vi "main.vi"(4 "force_read?":bool, 6 "custom_path":path, 7 "command":T1=enum."read_config", 8 "error in (no error)":errorcluster, 11 "config in":T2) -> (0 "error out":errorcluster, 3 "config out":T2)   [LabVIEW 2015, in "lv-config-json.lvlib"]
doc: "This VI is able to read/write configuration from all the associated modules defined in the master data cluster. It also acts as a functional global/data store in the event that no data has changed since the last write. It will self-initialize and well set an internal flag in the event an error is encountered when reading. If no command is provided, it will default to the read command."
uses:
  lv-config-json.lvlib
  public/_controls/configuration.ctl
  public/_controls/command.ctl
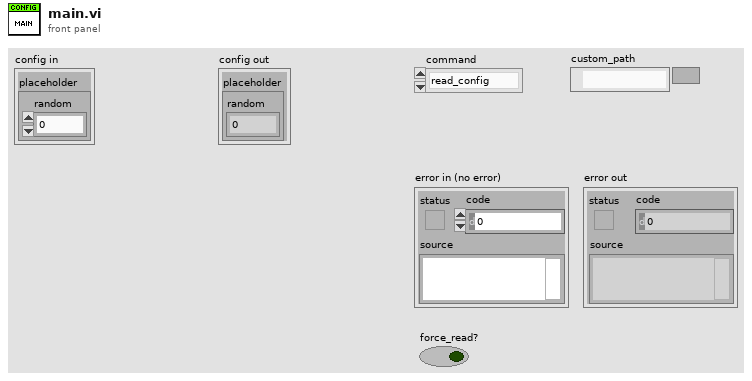
[diagram p1: front panel]
types:
  T1 = typedef "lv-config-json.lvlib/command.ctl" = enum16{"<commands>", "read_config", "write_config", "write_placeholder"}
  T2 = typedef "lv-config-json.lvlib/configuration.ctl" = cluster{"placeholder":cluster{"random":dbl}}
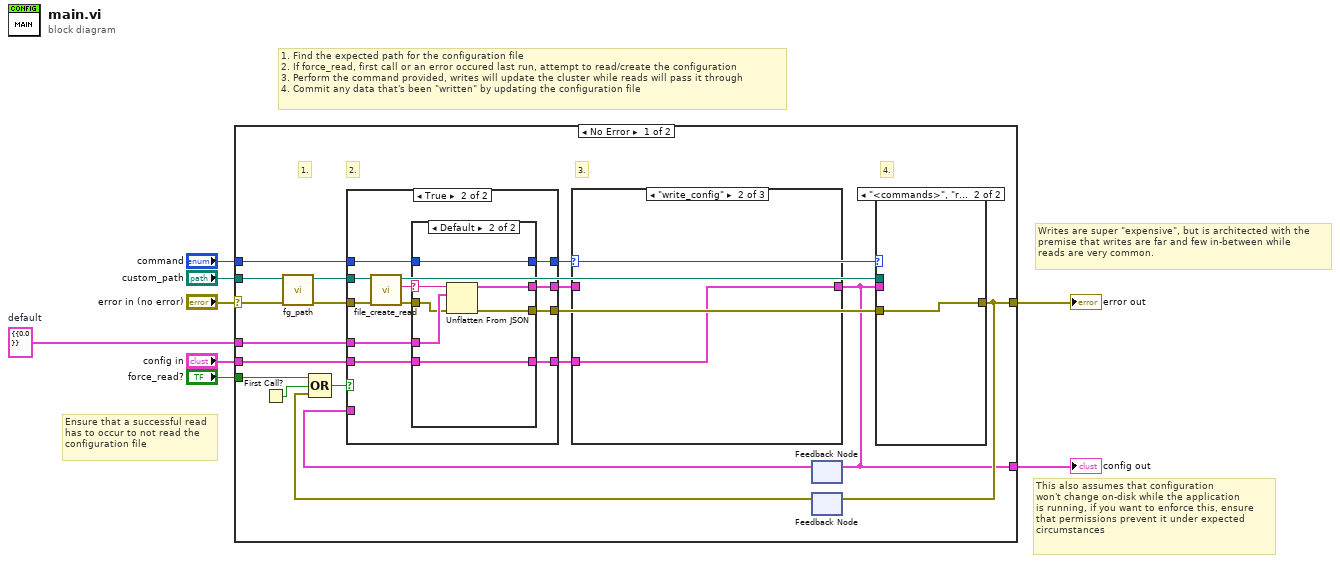
[diagram p0: block diagram]
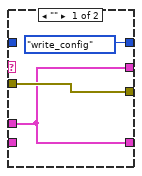
[diagram p3: hidden frame]
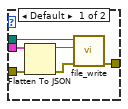
[diagram p4: hidden frame]
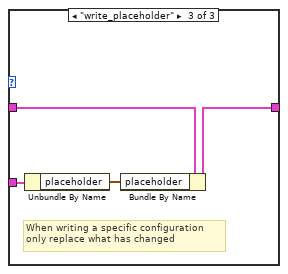
[diagram p6: hidden frame]
diagram:
  w1 = T2 {"placeholder"={"random"=0.0}}  # default
  # "This also assumes that configuration\nwon't change on-disk while the application\nis running, if you want to enforce this, ensure\nthat permissions prevent it under expected\ncircumstances"
  # "1. Find the expected path for the configuration file\n2. If force_read, first call or an error occured last run, attempt to read/create the configuration\n3. Perform the command provided, writes will update the cluster while reads will pass it through\n4. Commit any data that's been \"written\" by updating the configuration file"
  # "Writes are super \"expensive\", but is architected with the\npremise that writes are far and few in-between while\nreads are very common."
  # "Ensure that a successful read\nhas to occur to not read the\nconfiguration file"
  n1 = case shown="No Error" "error in (no error)" {
    selector: "error in (no error)" -> [w23 w65]
    tunnel: "command" -> [w13 _]
    tunnel: [w25 w65] -> w4
    tunnel: "config in" -> [w11 _]
    tunnel: "custom_path" -> [w22 _]
    tunnel: [w15 _] -> w3
    tunnel: "force_read?" -> [w20 _]
    tunnel: w1 -> [w16 _]
    frame No Error {
      # "4."
      # "3."
      # "2."
      # "1."
      n2 = First Call?() -> (First Call?: T/F=w21:bool)
      n3 = call "fg_path.vi"("error in (no error)"=w23, "custom_path"=w22) -> ("error out"=w17:errorcluster, "config_working"=w14:path)  [unwired: 8 in]
      n4 = feedback #1() -> (w18:T2)  [unwired: 1 in]
      n5 = feedback #2() -> (w24:errorcluster)  [unwired: 1 in]
      n6 = Compound Arithmetic op=OR(w20, w21, w24) -> (w19:bool)
      n7 = case shown="True" w19 {
        tunnel: w18 -> [w30 _]
        tunnel: w17 -> [w29 w39]
        tunnel: w14 -> [_ w40]
        tunnel: [w29 w37] -> w26
        tunnel: w16 -> [_ w41]
        tunnel: w13 -> [w28 w36]
        tunnel: [w28 w35] -> w12
        tunnel: w11 -> [w27 w34]
        tunnel: [w27 w33] -> w10
        tunnel: [w30 w32] -> w9
        frame False {
        }
        frame True {
          n8 = call "file_create_read.vi"("error in (no error)"=w39, "config_path"=w40) -> ("error out"=w38:errorcluster, "string"=w31:string)  [unwired: 8 in]
          n9 = case shown="Default" w31 {
            selector: w31 -> [_ w48]
            tunnel: w41 -> [w42 w51]
            tunnel: [w42 w50] -> w32
            tunnel: w38 -> [w44 w49]
            tunnel: [w44 w47] -> w37
            tunnel: w36 -> [_ w46]
            tunnel: [command."write_config" ("command") w46] -> w35
            tunnel: w34 -> [_ w45]
            tunnel: [w42 w45] -> w33
            frame "" {
            }
            frame Default {
              n10 = Unflatten From JSON(JSON string=w48, type and defaults=w51, error in (no error)=w49) -> (value=w50:T2, error out=w47:errorcluster)  [unwired: 4 in]
            }
          }
        }
      }
      n11 = case shown="\"write_config\"" w12 {
        tunnel: w10 -> [_ w60 w64]
        tunnel: [w59 w60 w61] -> w15
        tunnel: w9 -> [w59 _ w62]
        frame Default {
        }
        frame "write_config" {
        }
        frame "write_placeholder" {
          # "When writing a specific configuration\nonly replace what has changed"
          n12 = Unbundle By Name(w64) -> ("placeholder"=w63:cluster{"random":dbl})
          n13 = Bundle By Name(cluster=w62, "placeholder"=w63) -> (w61:T2)
        }
      }
      n14 = feedback-in #1(w15) -> ()
      n15 = case shown="\"<commands>\", \"read_config\"" w12 {
        tunnel: w15 -> [w54 _]
        tunnel: w26 -> [w55 w58]
        tunnel: [w52 w58] -> w25
        tunnel: w14 -> [w53 _]
        frame Default {
          n16 = Flatten To JSON(anything=w54, error in (no error)=w55) -> (JSON string=w57:string, 11:w56:errorcluster)  [unwired: 1 in]
          n17 = call "file_write.vi"("error in (no error)"=w56, "string"=w57, "config_path"=w53) -> ("error out"=w52:errorcluster)  [unwired: 8 in]
        }
        frame "<commands>", "read_config" {
        }
      }
      n18 = feedback-in #2(w25) -> ()
    }
    frame Error {
      # "If an error is wired in, be sure to skip over functionality to preserve the original error"
    }
  }
  "config out" <- w3
  "error out" <- w4
